vi "Main.Read DTC Values from VS.vi"(8 "error in":errorcluster, 11 "Simulated Addresses in":T1[](array[typedef]) {"Data"."DM1.Ref"."Data Reference" format="%.0x"; "Data"."DM1.Enable.Ref"."Data Reference" format="%.0x"; "Data"."DM2.Ref"."Data Reference" format="%.0x"; "Data"."DM2.Enable.Ref"."Data Reference" format="%.0x"}) -> (0 "error out":errorcluster, 3 "Simulated Addresses out":T1[](array[typedef]) {"Data"."DM1.Ref"."Data Reference" format="%.0x"; "Data"."DM1.Enable.Ref"."Data Reference" format="%.0x"; "Data"."DM2.Ref"."Data Reference" format="%.0x"; "Data"."DM2.Enable.Ref"."Data Reference" format="%.0x"})   [LabVIEW 2023, in "J1939 Addon Engine.lvlib"]
uses:
  J1939 Addon Engine.lvlib
  Types/Engine.DTC Settings.ctl
  Addon Shared/Types/Compiled Simulated Settings.ctl
  <vilib>/NI VeriStand/Custom Device API/Block Data Reference.ctl
  <vilib>/NI VeriStand/Custom Device API/Data Reference.ctl
  Types/Engine.DTC FIFOs.ctl
  <vilib>/NI VeriStand/Custom Device API/Global Data Refs.vi
  <vilib>/NI VeriStand/Custom Device API/Custom Device API.lvlib
  Addon Shared/J1939 Addon Shared.lvlib
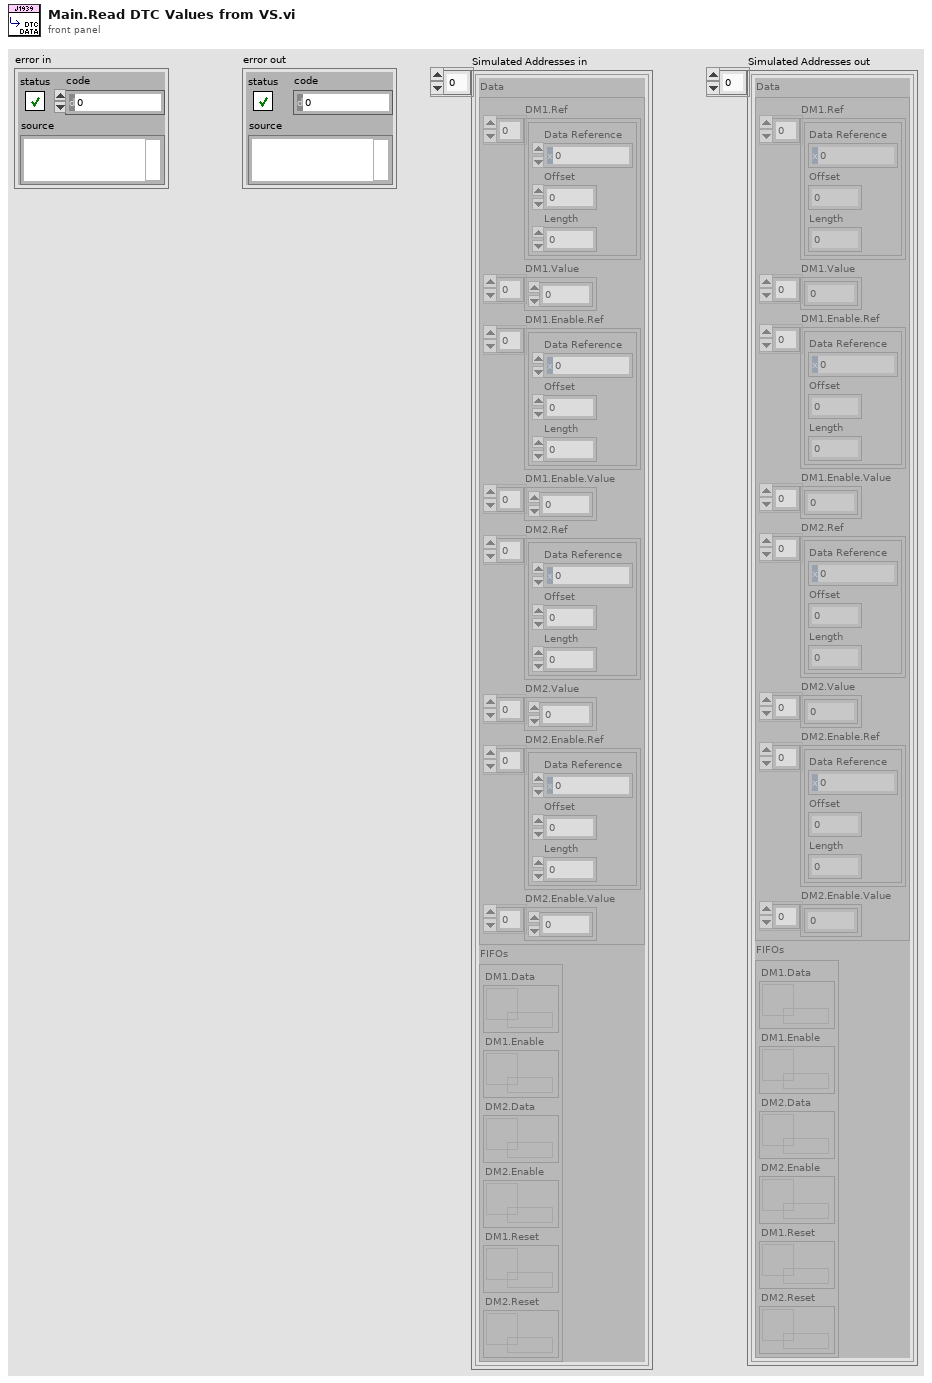
[diagram p1: front panel]
types:
  T1 = typedef "J1939 Addon Engine.lvlib/Engine.DTC Settings.ctl" = cluster{"Data":T2, "FIFOs":T5}
  T2 = typedef "J1939 Addon Shared.lvlib/Compiled Simulated Settings.ctl" = cluster{"DM1.Ref":T3[], "DM1.Value":dbl[], "DM1.Enable.Ref":T3[], "DM1.Enable.Value":dbl[], "DM2.Ref":T3[], "DM2.Value":dbl[], "DM2.Enable.Ref":T3[], "DM2.Enable.Value":dbl[]}
  T3 = typedef "Custom Device API.lvlib/Block Data Reference.ctl" = cluster{"Data Reference":T4, "Offset":u64, "Length":u64}
  T4 = typedef "Custom Device API.lvlib/Data Reference.ctl" = i32
  T5 = typedef "J1939 Addon Engine.lvlib/Engine.DTC FIFOs.ctl" = cluster{"DM1.Data":refnum<k33>, "DM1.Enable":refnum<k33>, "DM2.Data":refnum<k33>, "DM2.Enable":refnum<k33>, "DM1.Reset":refnum<k33>, "DM2.Reset":refnum<k33>}
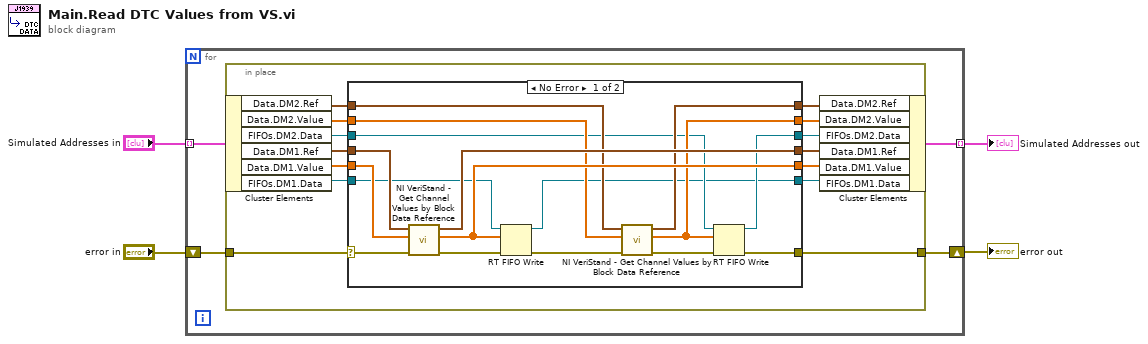
[diagram p0: block diagram]
diagram:
  n1 = for {
    tunnel: [w7] -> w1 mode=indexing
    tunnel: "Simulated Addresses in" -> [w5] mode=indexing
    shift-right: [w8] -> w4
    shift-left: "error in" -> [w6]
    n2 = in-place {
      in-place-border: [w22] -> w8
      in-place-border: w6 -> [w19]
      n3 = in-place-cluster #1(w5) -> ("Data.DM2.Ref"=w15:T3[], "Data.DM2.Value"=w14:dbl[], "FIFOs.DM2.Data"=w13:refnum<k33>, "Data.DM1.Ref"=w21:T3[], "Data.DM1.Value"=w18:dbl[], "FIFOs.DM1.Data"=w16:refnum<k33>)
      n4 = case shown="No Error" w19 {
        selector: w19 -> [w39 w46]
        tunnel: [w27 w46] -> w22
        tunnel: [w34 w44] -> w17
        tunnel: w21 -> [w37 w45]
        tunnel: [w36 w45] -> w20
        tunnel: w18 -> [w35 w44]
        tunnel: w16 -> [w24 w40]
        tunnel: w15 -> [w31 w41]
        tunnel: w14 -> [w30 w42]
        tunnel: w13 -> [w26 w43]
        tunnel: [w25 w43] -> w12
        tunnel: [w23 w40] -> w11
        tunnel: [w29 w42] -> w10
        tunnel: [w28 w41] -> w9
        frame No Error {
          n5 = call <vilib>:"NI VeriStand - Get Channel Values by Block Data Reference.vi"("error in (no error)"=w39, "Values Array in"=w35, "Block Data Ref"=w37) -> ("error out"=w38:errorcluster, "Values Array out"=w34:dbl[], "Block Data Ref dup"=w36:T3[])  [unwired: 6 in]
          n6 = RT FIFO Write(0:w24, 1:w34, 3:w38) -> (8:w23:refnum<k33>, 11:w32:errorcluster)  [unwired: 2 in, 2 out]
          n7 = call <vilib>:"NI VeriStand - Get Channel Values by Block Data Reference.vi"("error in (no error)"=w32, "Values Array in"=w30, "Block Data Ref"=w31) -> ("error out"=w33:errorcluster, "Values Array out"=w29:dbl[], "Block Data Ref dup"=w28:T3[])  [unwired: 6 in]
          n8 = RT FIFO Write(0:w26, 1:w29, 3:w33) -> (8:w25:refnum<k33>, 11:w27:errorcluster)  [unwired: 2 in, 2 out]
        }
        frame Error {
        }
      }
      n9 = in-place-cluster #1("Data.DM2.Ref"=w9, "Data.DM2.Value"=w10, "FIFOs.DM2.Data"=w12, "Data.DM1.Ref"=w20, "Data.DM1.Value"=w17, "FIFOs.DM1.Data"=w11) -> (w7:T1)
    }
  }
  "error out" <- w4
  "Simulated Addresses out" <- w1
